vi "THERM3dll.vi"(8 "error in (no error)":errorcluster, 11 "Inputs":cluster{"t":dbl, "D":dbl, "z":dbl[]}) -> (0 "error out":errorcluster, 3 "Outputs":T1)   [LabVIEW 2021]
doc: "subroutine THERM3dll(t, D, z, xkappa, beta, xisenk, xkt, betas, bs, xkkt, thrott, pi, spht)\n\nCompute miscellaneous thermodynamic properties. See warning in suroutines THERM or ALLPROPS.\n\nINPUTS:\nt --Temperature [K]\nD -- Molar density [mol/L]\nz -- Composition (array of mole fractions)\n\nOUTPUTS:\nxkappa -- Isothermal compressibility [1/kPa]\nbeta -- Volume expansivity [1/K]\nxisenk -- Isentropic expansion coefficient [-]\nxkt -- Isothermal expansion coefficient [-]\nbetas -- Adiabatic compressibility [1/kPa]\nbs -- Adiabatic bulk modulus [kPa]\nxkkt -- Isothermal bulk modulus [kPa]\nthrott -- Isothermal throttling coefficient [L/mol]\npi -- Internal pressure [kPa]\nspht -- Specific heat input [J/mol]"
uses:
  REFPROP.dll
panel:
  # "REFPROP-THERM3dll.vi"
  # "void  THERM3dll(double *t, double *D, double *z, double *kappa, double *beta, double *xisenk, double *xkt, double *betas, double *bs, double *xkkt, double *thrott, double *pi, double *spht)"
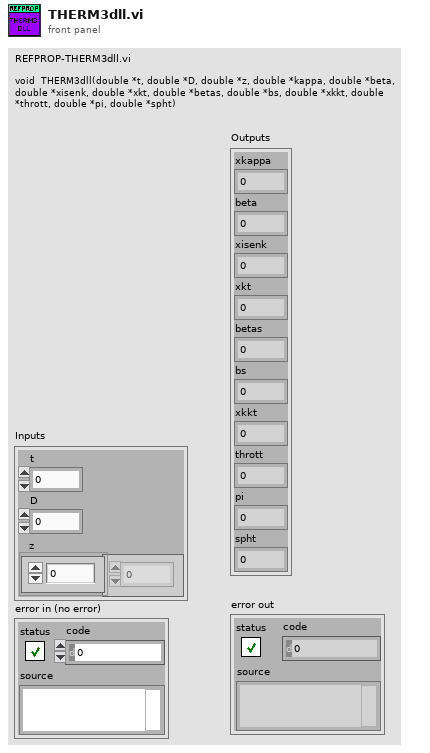
[diagram p1: front panel]
types:
  T1 = cluster{"xkappa ":dbl, "beta ":dbl, "xisenk ":dbl, "xkt ":dbl, "betas":dbl, "bs":dbl, "xkkt ":dbl, "thrott":dbl, "pi":dbl, "spht":dbl}
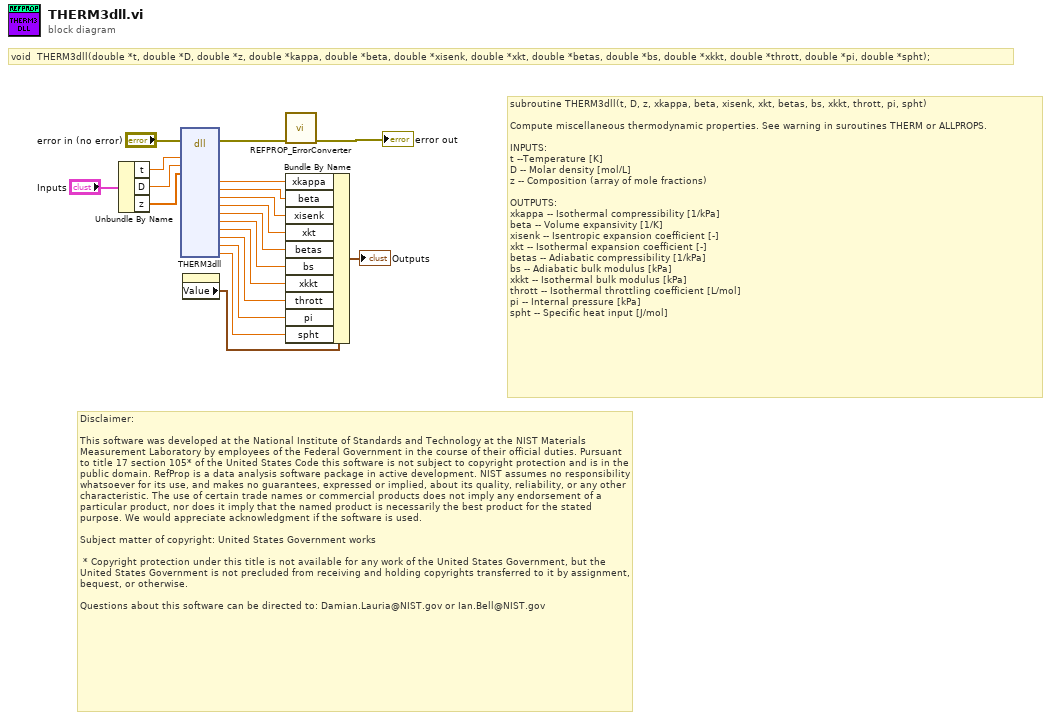
[diagram p0: block diagram]
diagram:
  # "Disclaimer:\n\nThis software was developed at the National Institute of Standards and Technology at the NIST Materials Measurement Laboratory by employees of the Federal Government in the course of their official duties. Pursuant to title 17 section 105* of the United States Code this software is not subject to copyright protection and is in the public domain. RefProp is a data analysis software package in active development. NIST assumes no responsibility whatsoever for its use, and makes no guarantees, expressed or implied, about its quality, reliability, or any other characteristic. The use of certain trade names or commercial products does not imply any endorsement of a particular product, nor does it imply that the named product is necessarily the best product for the stated purpose. We would appreciate acknowledgment if the software is used.\n \nSubject matter of copyright: United States Government works\n  \n * Copyright protection under this title is not available for any work of the United States Government, but the United States Government is not precluded from receiving and holding copyrights transferred to it by assignment, bequest, or otherwise.\n\nQuestions about this software can be directed to: Damian.Lauria@NIST.gov or Ian.Bell@NIST.gov"
  # "void  THERM3dll(double *t, double *D, double *z, double *kappa, double *beta, double *xisenk, double *xkt, double *betas, double *bs, double *xkkt, double *thrott, double *pi, double *spht);"
  # "subroutine THERM3dll(t, D, z, xkappa, beta, xisenk, xkt, betas, bs, xkkt, thrott, pi, spht)\n\nCompute miscellaneous thermodynamic properties. See warning in suroutines THERM or ALLPROPS.\n\nINPUTS:\nt --Temperature [K]\nD -- Molar density [mol/L]\nz -- Composition (array of mole fractions)\n\nOUTPUTS:\nxkappa -- Isothermal compressibility [1/kPa]\nbeta -- Volume expansivity [1/K]\nxisenk -- Isentropic expansion coefficient [-]\nxkt -- Isothermal expansion coefficient [-]\nbetas -- Adiabatic compressibility [1/kPa]\nbs -- Adiabatic bulk modulus [kPa]\nxkkt -- Isothermal bulk modulus [kPa]\nthrott -- Isothermal throttling coefficient [L/mol]\npi -- Internal pressure [kPa]\nspht -- Specific heat input [J/mol]"
  n1 = Unbundle By Name("Inputs") -> ("t"=w15:dbl, "D"=w14:dbl, "z"=w13:dbl[])
  n2 = dll-call lib="C:/Users/lauria/OneDrive - National Institute of Standards and Technology (NIST)/LabVIEW Projects/7 REFPROP/REFPROP-wrappers-master/REFPROP-wrappers-master/wrappers/Labview/REFPROP/REFPROP.*" fn="THERM3dll"(error in="error in (no error)", "t"=w15, "D"=w14, "z"=w13) -> (error out=w19:errorcluster, "kappa"=w10:dbl, "beta"=w9:dbl, "xisenk"=w8:dbl, "xkt"=w7:dbl, "betas"=w6:dbl, "bs"=w5:dbl, "xkkt"=w4:dbl, "thrott"=w3:dbl, "pi"=w2:dbl, "spht"=w1:dbl)  [unwired: 16 in, 1 out]
  n3 = property on="Outputs" class="Clust (strict)"() -> ("Value"=w12:T1)  [unwired: 2 in, 2 out]
  n4 = call "REFPROP_ErrorConverter.vi"("error in (no error)"=w19) -> ("error out"=→"error out":errorcluster)  [unwired: 10 in]
  n5 = Bundle By Name(cluster=w12, "xkappa"=w10, "beta"=w9, "xisenk"=w8, "xkt"=w7, "betas"=w6, "bs"=w5, "xkkt"=w4, "thrott"=w3, "pi"=w2, "spht"=w1) -> (→"Outputs":T1)
